vi "Read Speaker State CMD.vi"(8 "error in (no error)":errorcluster, 11 "PAS in":refnum<class "PAS.lvclass">) -> (0 "error out":errorcluster, 2 "PAS Library.lvlib:Change Speaker State CMD":refnum<class "Change Speaker State CMD.lvclass">, 3 "PAS out":refnum<class "PAS.lvclass">)   [LabVIEW 2016, in "PAS Library.lvlib" / "PAS.lvclass"]
uses:
  PAS.lvclass
  Commands/Change Speaker State CMD/Change Speaker State CMD.lvclass
  PAS.lvclass/PAS.ctl
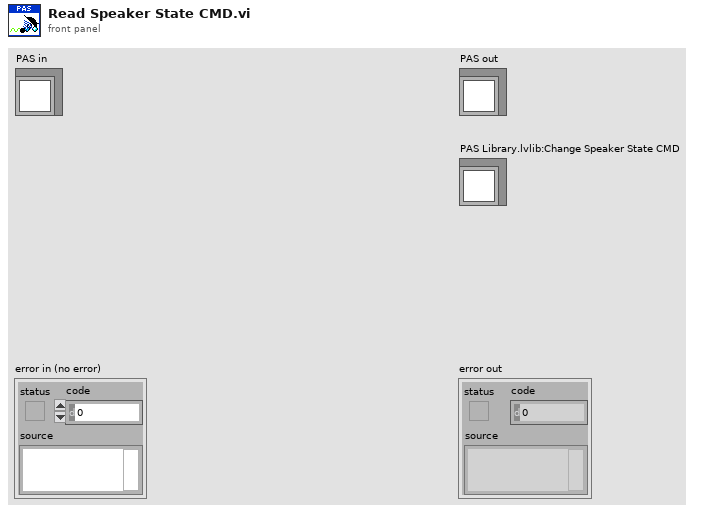
[diagram p1: front panel]
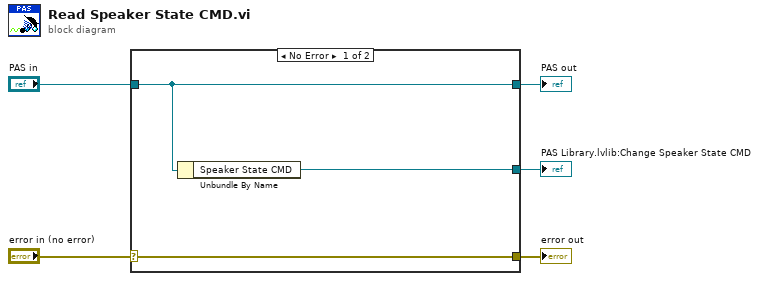
[diagram p0: block diagram]
diagram:
  n1 = case shown="No Error" "error in (no error)" {
    selector: "error in (no error)" -> [w8 w9]
    tunnel: [w8 w9] -> w4
    tunnel: [w7 w10] -> w2
    tunnel: "PAS in" -> [w7 w10]
    tunnel: [w6 _] -> w1
    frame No Error {
      n2 = Unbundle By Name(w7) -> ("Speaker State CMD"=w6:refnum<class "Change Speaker State CMD.lvclass">)
    }
    frame Error {
    }
  }
  "error out" <- w4
  "PAS out" <- w2
  "PAS Library.lvlib:Change Speaker State CMD" <- w1
